vi "读取版本号.vi"() -> ()   [LabVIEW 2020]
uses:
  Libraries/ZLG_CAN/ZLG_CAN.lvlib
panel:
  in  "产品型号":u16(ring) items=["R92A", "R527", "R538"]
  out "硬件版本":string
  out "软件版本":string
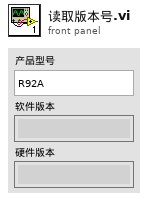
[diagram p1: front panel]
types:
  T1 = cluster{"[0]":u8, "[1]":u8, "[2]":u8, "[3]":u8, "[4]":u8, "[5]":u8, "[6]":u8, "[7]":u8}[]
  T2 = typedef "ZLG_CAN.lvlib/Recive_Wait (Reply Payload)--cluster.ctl" = cluster{"Can_Receive":T3[], "Recive_Wait_error":errorcluster}
  T3 = typedef "ZLG_CAN.lvlib/CAN_OBJ_R.ctl" = cluster{"ID":u32, "TimeStamp":u32, "TimeFlag":u8, "SendType":u8, "RemoteFlag":u8, "ExternFlag":u8, "DataLen":u8, "数值":u8, "数值":u8, "数值":u8, "数值":u8, "数值":u8, "数值":u8, "数值":u8, "数值":u8, "数值":u8, "数值":u8, "数值":u8}
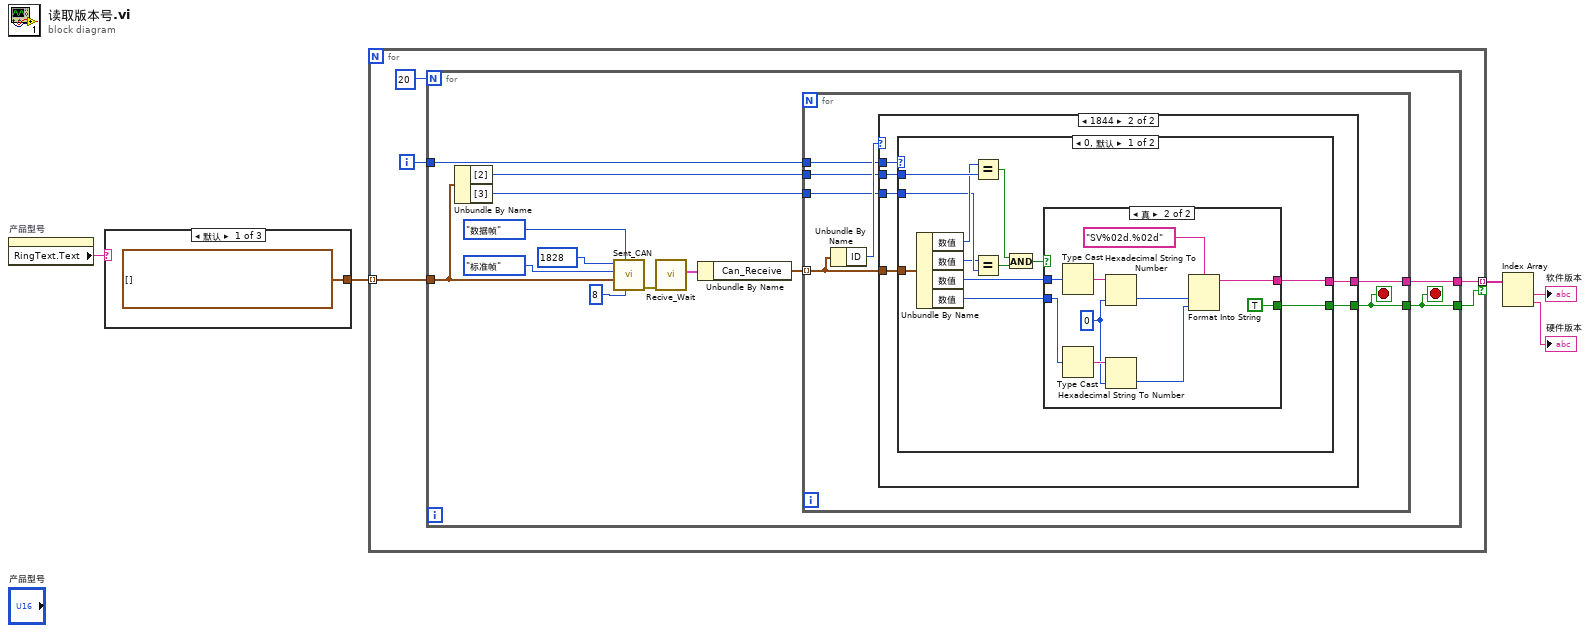
[diagram p0: block diagram]
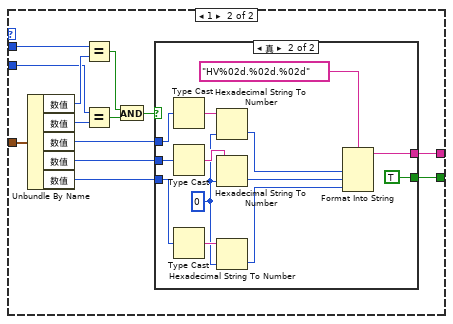
[diagram p4: hidden frame]
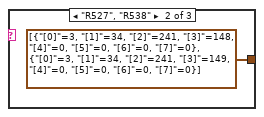
[diagram p6: hidden frame]
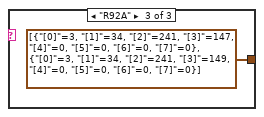
[diagram p7: hidden frame]
diagram:
  n1 = property on="产品型号" class="Ring (严格)"() -> ("RingText.Text"=w1:string)  [unwired: 2 in, 2 out]
  n2 = case shown="默认" w1 {
    tunnel: [T1 [] T1 [{"[0]"=3, "[1]"=34, "[2]"=241, "[3]"=148, "[4]"=0, "[5]"=0, "[6]"=0, "[7]"=0}, {"[0]"=3, "[1]"=34, "[2]"=241, "[3]"=149, "[4]"=0, "[5]"=0, "[6]"=0, "[7]"=0}] T1 [{"[0]"=3, "[1]"=34, "[2]"=241, "[3]"=147, "[4]"=0, "[5]"=0, "[6]"=0, "[7]"=0}, {"[0]"=3, "[1]"=34, "[2]"=241, "[3]"=149, "[4]"=0, "[5]"=0, "[6]"=0, "[7]"=0}]] -> w5
    frame Default {
    }
    frame "R527", "R538" {
    }
    frame "R92A" {
    }
  }
  n3 = for {
    tunnel: w5 -> [w13] mode=indexing
    tunnel: [w10] -> w4 mode=indexing if=w9
    i -> [w11]
    n4 = for {
      N: 20 -> [_]
      tunnel: w13 -> [w17]
      tunnel: w11 -> [w25]
      tunnel: [w24] -> w10
      tunnel: [w14] -> w9
      stop <- w14 stop-if-true
      n5 = Unbundle By Name(w17) -> ("[2]"=w16:u8, "[3]"=w15:u8)
      n6 = call "Sent_CAN.vi"("帧长度"=u8 8, "帧类型"=enum16{"数据帧", "远程帧"}."数据帧" ("帧格式"), "帧数据"=w17, "帧格式"=enum8{"标准帧", "扩展帧"}."标准帧" ("帧类型"), "ID"=u32 1828) -> ("error out"=w19:errorcluster)  [unwired: 6 in]
      n7 = call "Recive_Wait.vi"("error in (no error)"=w19) -> ("Reply Payload"=w18:T2)  [unwired: 8 in, 2 out]
      n8 = Unbundle By Name(w18) -> ("Can_Receive"=w26:T3[])
      n9 = for {
        tunnel: w26 -> [w32] mode=indexing
        tunnel: w25 -> [w31]
        tunnel: [w30] -> w24
        tunnel: w16 -> [w29]
        tunnel: w15 -> [w28]
        tunnel: [w27] -> w14
        stop <- w27 stop-if-true
        n10 = Unbundle By Name(w32) -> ("ID"=w33:u32)
        n11 = case shown="1844" w33 {
          tunnel: w32 -> [_ w39]
          tunnel: [_ w38] -> w30
          tunnel: [_ w34] -> w27
          tunnel: w31 -> [_ w37]
          tunnel: w29 -> [_ w36]
          tunnel: w28 -> [_ w35]
          frame 0, Default {
          }
          frame 1844 {
            n12 = case shown="0, 默认" w37 {
              tunnel: w39 -> [w51 w74]
              tunnel: [w48 w73] -> w38
              tunnel: w36 -> [w47 w66]
              tunnel: w35 -> [w45 w65]
              tunnel: [w40 w62] -> w34
              frame 0, Default {
                n13 = Unbundle By Name(w51) -> ("数值"=w46:u8, "数值"=w44:u8, "数值"=w50:u8, "数值"=w49:u8)
                n14 = Equal?(x=w46, y=w47) -> (x = y?=w43:bool)
                n15 = Equal?(x=w44, y=w45) -> (x = y?=w42:bool)
                n16 = And(x=w43, y=w42) -> (x .and. y?=w41:bool)
                n17 = case shown="真" w41 {
                  tunnel: w50 -> [_ w59]
                  tunnel: w49 -> [_ w58]
                  tunnel: [_ w54] -> w48
                  tunnel: [_ TRUE] -> w40
                  frame False {
                  }
                  frame True {
                    w53 = u8 0 ("默认(0 U32)")
                    n18 = Type Cast(x=w59) -> (*(type *) &x=w61:string)  [unwired: 1 in]
                    n19 = Type Cast(x=w58) -> (*(type *) &x=w60:string)  [unwired: 1 in]
                    n20 = Hexadecimal String To Number(string=w61, default (0uL)=w53) -> (number=w56:u8)  [unwired: 1 in, 1 out]
                    n21 = Hexadecimal String To Number(string=w60, default (0uL)=w53) -> (number=w55:u8)  [unwired: 1 in, 1 out]
                    n22 = Format Into String(format string="SV%02d.%02d" ("格式字符串"), w56, w55) -> (resulting string=w54:string)  [unwired: 2 in, 1 out]
                  }
                }
              }
              frame 1 {
                n23 = Unbundle By Name(w74) -> ("数值"=w67:u8, "数值"=w64:u8, "数值"=w72:u8, "数值"=w71:u8, "数值"=w70:u8)
                n24 = Equal?(x=w66, y=w67) -> (x = y?=w69:bool)
                n25 = Equal?(x=w65, y=w64) -> (x = y?=w68:bool)
                n26 = And(x=w69, y=w68) -> (x .and. y?=w63:bool)
                n27 = case shown="真" w63 {
                  tunnel: [_ w79] -> w73
                  tunnel: w72 -> [_ w78]
                  tunnel: w71 -> [_ w77]
                  tunnel: w70 -> [_ w76]
                  tunnel: [_ TRUE] -> w62
                  frame False {
                  }
                  frame True {
                    w81 = u8 0 ("默认(0 U32)")
                    n28 = Type Cast(x=w78) -> (*(type *) &x=w85:string)  [unwired: 1 in]
                    n29 = Type Cast(x=w77) -> (*(type *) &x=w84:string)  [unwired: 1 in]
                    n30 = Type Cast(x=w76) -> (*(type *) &x=w86:string)  [unwired: 1 in]
                    n31 = Hexadecimal String To Number(string=w85, default (0uL)=w81) -> (number=w83:u8)  [unwired: 1 in, 1 out]
                    n32 = Hexadecimal String To Number(string=w84, default (0uL)=w81) -> (number=w82:u8)  [unwired: 1 in, 1 out]
                    n33 = Hexadecimal String To Number(string=w86, default (0uL)=w81) -> (number=w87:u8)  [unwired: 1 in, 1 out]
                    n34 = Format Into String(format string="HV%02d.%02d.%02d" ("格式字符串"), w83, w82, w87) -> (resulting string=w79:string)  [unwired: 2 in, 1 out]
                  }
                }
              }
            }
          }
        }
      }
    }
  }
  n35 = Index Array(array=w4) -> (element #1=→"软件版本":string, element #2=→"硬件版本":string)  [unwired: 2 in]
